vi "SendEvent(SubVI).vi"(8 "error in (no error)":errorcluster, 9 "Data":variant, 10 "Command":T2=enum."Idle", 11 "ID":T1) -> (0 "Error Out":errorcluster)   [LabVIEW 2017]
uses:
  TypeDefs/FGV_Enum.ctl
  MainFrameLib.lvlib
  TypeDefs/Command_Enum.ctl
  TypeDefs/DataCluster.ctl
  TypeDefs/ID_Enum.ctl
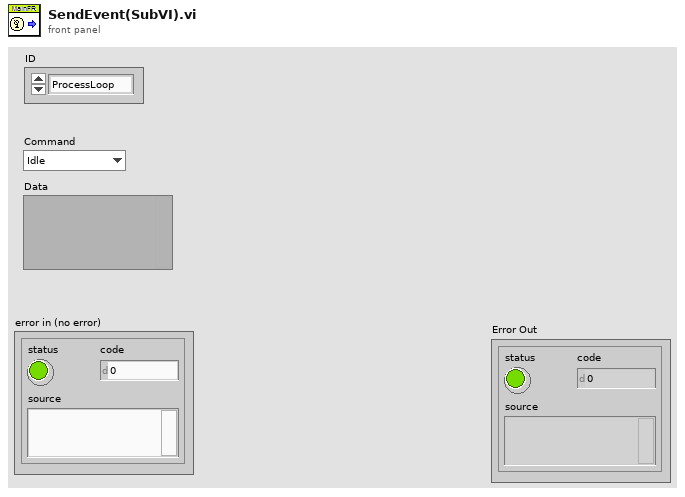
[diagram p1: front panel]
types:
  T1 = typedef "ID_Enum.ctl" = enum16{"ProcessLoop", "UILoop"}
  T2 = typedef "MainFrameLib.lvlib/Command_Enum.ctl" = enum16{"GetSRNotes", "DisplayAEStats", "InWork&Neglected", "RemapAENames", "ClearFolder", "UpdateReportsList", "ExcelReports", "TeamStats", "LoadReport", "WaitOnReport", "RequestReport", "Error", "Idle", "Initialize", "ScreenPop", "ClipboardCopy", "Shutdown"}
  T3 = typedef "MainFrameLib.lvlib/DataCluster.ctl" = cluster{"Command":T2, "Data":variant}
  T4 = typedef "MainFrameLib.lvlib/FGV_Enum.ctl" = enum16{"Close", "GetEventRefs", "Set"}
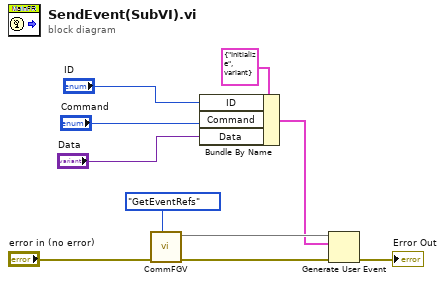
[diagram p0: block diagram]
diagram:
  n1 = call "CommFGV.vi"(7:FGV_Enum."GetEventRefs", "Error In"="error in (no error)") -> ("error out"=w10:errorcluster, 3:w4)  [unwired: 8 in]
  n2 = Bundle By Name(cluster=T3 {"Command"=enum."Initialize", "Data"=variant} ("event data"), "ID"="ID", "Command"="Command", "Data"="Data") -> (w2:T3)
  n3 = Generate User Event(user event=w4, event data cluster=w2, error in=w10) -> (error out=→"Error Out":errorcluster)  [unwired: 1 in, 1 out]
